vi "Open valves.vi"() -> ()   [LabVIEW 2014]
uses:
  <vilib>/Platform/TimedLoop/XDataNode/timing_clust.ctl
  <vilib>/Platform/TimedLoop/XDataNode/nitl_modes.ctl
  <vilib>/Platform/TimedLoop/XDataNode/wakeup.ctl
  <vilib>/DAQmx/write.llb/DAQmx Write (Digital 1D Bool NChan 1Samp 1Line).vi
  <vilib>/platform/TimedLoop/XDataNode/XDataNode.xnode
  <vilib>/Platform/TimedLoop/XDataNode/XDNodeRunTimeDep.lvlib
panel:
  in  "Cycle #":i32=80
  in  "Stop program":bool
  in  "Cycle duration (us)":i64=500
  in  "Open valves":bool
  in  "Close valves":bool
  out "error out":errorcluster
  # "Reward: 500us, 70 cycles"
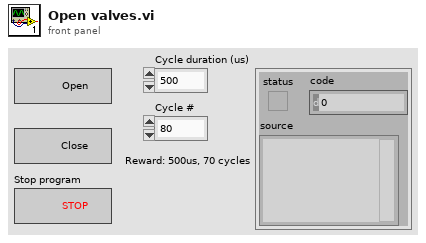
[diagram p1: front panel]
types:
  T1 = typedef "XDNodeRunTimeDep.lvlib/timing_clust.ctl" = cluster{"Expected End [f-1]":u64, "Actual End [f-1]":u64, "Finished Late? [f-1]":bool, "Expected End [i-1]":u64, "Actual End [i-1]":u64, "Finished Late? [i-1]":bool, "Expected Start [i]":u64, "Actual Start [i]":u64, "Expected Start [f]":u64, "Actual Start [f]":u64, "Source Name":string, "Structure Name":string, "Period":i64, "Deadline":i64, "Offset":i64, "Start":i64, "Priority":i32, "Timeout":i32, "Mode":T2, "Wakeup Reason":T3, "Error":errorcluster, "Source Type":string, "Secondary Source Type":string, "Global End Time":u64, "Global Start Time":u64, "Frame Duration":u64, "Iteration Duration":u64, "Assigned CPU":i32, "I/O Scan Engine Mode":u32}
  T2 = typedef "XDNodeRunTimeDep.lvlib/nitl_modes.ctl" = enum32{"No Change", "Process missed periods, maintain original phase", "Discard missed periods, maintain original phase", "Process missed periods, ignore original phase", "Discard missed periods, ignore original phase"}
  T3 = typedef "XDNodeRunTimeDep.lvlib/wakeup.ctl" = enum32{"Normal", "Aborted", "Asynchronous wakeup", "Timing source error", "Timed loop error", "Timeout"}
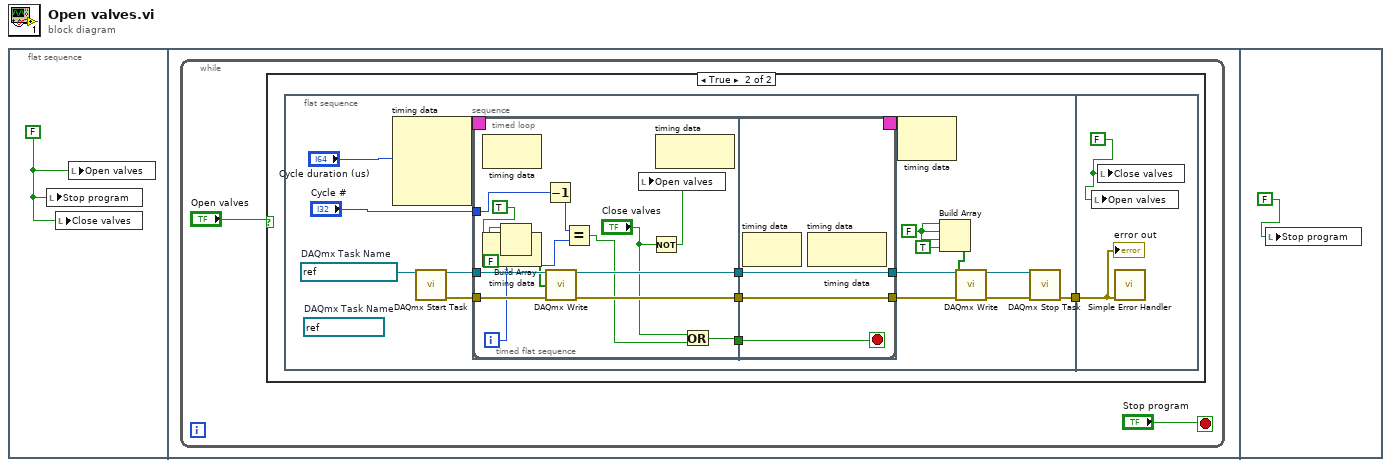
[diagram p0: block diagram]
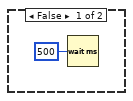
[diagram p2: hidden frame]
diagram:
  n1 = flat-sequence {
    frame #0 {
      w1 = FALSE
      n2 = local write "Stop program"(w1) -> ()
      n3 = local write "Close valves"(w1) -> ()
      n4 = local write "Open valves"(w1) -> ()
    }
    frame #1 {
      n5 = while {
        stop <- "Stop program" stop-if-true
        n6 = case shown="True" "Open valves" {
          frame False {
            n7 = Wait (ms)(milliseconds to wait=u32 500) -> ()  [unwired: 1 out]
          }
          frame True {
            n8 = flat-sequence {
              tunnel: [w11] -> w5
              tunnel: w5 -> [w62]
              frame #0 {
                (unwired) refnum<k21> "ExciseValves"  # DAQmx Task Name
                w7 = FALSE
                w18 = refnum<k21> "digitWrite"  # DAQmx Task Name
                n9 = node-c288("Cycle duration (us)") -> (w20:T1)  [unwired: 3 in]
                n10 = call <vilib>:"DAQmx Start Task.vi"("task/channels in"=w18) -> ("task out"=w17:refnum<k21>, "error out"=w16:errorcluster)  [unwired: 13 in]
                n11 = timed-loop {
                  timing: w20 -> [_]
                  timing-out: [_] -> w19
                  tunnel: w17 -> [w25]
                  tunnel: w16 -> [w24]
                  tunnel: [w23] -> w15
                  tunnel: [w22] -> w13
                  tunnel: "Cycle #" -> [w21]
                  i -> [w36]
                  stop <- w50 stop-if-true
                  n12 = timed-sequence {
                    timing: _ -> [_]
                    timing-out: _ -> [_]
                    tunnel: w25 -> [w33]
                    tunnel: w24 -> [w32]
                    tunnel: [w31] -> w23
                    tunnel: [w30] -> w22
                    tunnel: w21 -> [w26]
                    n13 = timed-flat-sequence {
                      tunnel: w33 -> [w47]
                      tunnel: w32 -> [w46]
                      tunnel: [w45] -> w29
                      tunnel: [w44] -> w28
                      tunnel: [w41] -> w27
                      tunnel: w26 -> [w37]
                      tunnel: [w51] -> w30
                      tunnel: [w52] -> w31
                      tunnel: w29 -> [w52]
                      tunnel: w28 -> [w51]
                      tunnel: w27 -> [w50]
                      frame #0 {
                        w34 = TRUE
                        n14 = node-c288() -> ()  [unwired: 1 in, 1 out]
                        n15 = Build Array(FALSE, w34, w34, w34) -> (w43:bool[])
                        n16 = Decrement(x=w37) -> (x-1=w38:i32)
                        n17 = call-poly <vilib>:"DAQmx Write.vi"("task/channels in"=w47, "data"=w43, "error in"=w46) -> ("task out"=w45:refnum<k21>, "error out"=w44:errorcluster)  [unwired: 10 in, 1 out]
                        n18 = Equal?(x=w38, y=w36) -> (x = y?=w39:bool)
                        n19 = Not(x="Close valves") -> (.not. x?=w42:bool)
                        n20 = local write "Open valves"(w42) -> ()
                        n21 = node-c288() -> ()  [unwired: 1 in, 1 out]
                        n22 = Or(x="Close valves", y=w39) -> (x .or. y?=w41:bool)
                      }
                      frame #1 {
                        n23 = node-c288() -> ()  [unwired: 1 in, 1 out]
                        n24 = node-c288() -> ()  [unwired: 1 in, 1 out]
                      }
                    }
                  }
                  n25 = node-c288() -> ()  [unwired: 1 in, 1 out]
                  n26 = node-c288() -> ()  [unwired: 1 in, 1 out]
                }
                n27 = node-c288(w19) -> ()  [unwired: 1 out]
                n28 = Build Array(w7, w7, w7, TRUE ("element")) -> (w10:bool[])
                n29 = call-poly <vilib>:"DAQmx Write.vi"("task/channels in"=w15, "data"=w10, "error in"=w13) -> ("task out"=w14:refnum<k21>, "error out"=w12:errorcluster)  [unwired: 10 in, 1 out]
                n30 = call <vilib>:"DAQmx Stop Task.vi"("task/channels in"=w14, "error in"=w12) -> ("error out"=w11:errorcluster)  [unwired: 12 in, 1 out]
              }
              frame #1 {
                w61 = FALSE
                n31 = local write "Open valves"(w61) -> ()
                n32 = local write "Close valves"(w61) -> ()
                n33 = call <vilib>:"Simple Error Handler.vi"("error in (no error)"=w62) -> ()  [unwired: 4 in, 5 out]
                "error out" <- w62
              }
            }
          }
        }
      }
    }
    frame #2 {
      n34 = local write "Stop program"(FALSE) -> ()
    }
  }
